vi "APC_9056_NI9214conf.vi"() -> (5 "channels name out":string[](array[string])=["WF-TT-001", "O2-TT-001", "AR-TT-001", "NG-TT-001", "NGDI-TT-001", "WF-TT-002 ", "WF-TT-003", "WF-TT-004", "WF-TT-007", "PC-TT-001", "PC-TT-002", "PC-TT-003", "PC-TT-004", "PC-TT-005", "PC-TT-006", "EC-TT-001", "EC-TT-002", "SW-TT-001", "SW-TT-002", "SW-TT-003", "SW-TT-004", "SW-TT-005", "SW-TT-006", "SW-TT-007", "SW-TT-008", "SW-TT-009", "EO-TT-001", "EO-TT-002", "NI9214b_13", "NI9214b_14", "NI9214b_15", "NI9214b_16"])   [LabVIEW 2020]
panel:
  in  "NI9214_B":string[](array[string])=["EC-TT-002", "SW-TT-001", "SW-TT-002", "SW-TT-003", "SW-TT-004", "SW-TT-005", "SW-TT-006", "SW-TT-007", "SW-TT-008", "SW-TT-009", "EO-TT-001", "EO-TT-002", "NI9214b_13", "NI9214b_14", "NI9214b_15", "NI9214b_16"]
  in  "NI9214_A":string[](array[string])=["WF-TT-001", "O2-TT-001", "AR-TT-001", "NG-TT-001", "NGDI-TT-001", "WF-TT-002 ", "WF-TT-003", "WF-TT-004", "WF-TT-007", "PC-TT-001", "PC-TT-002", "PC-TT-003", "PC-TT-004", "PC-TT-005", "PC-TT-006", "EC-TT-001"]
  # "NI9214"
  # "_degC is added automatically to all channels"
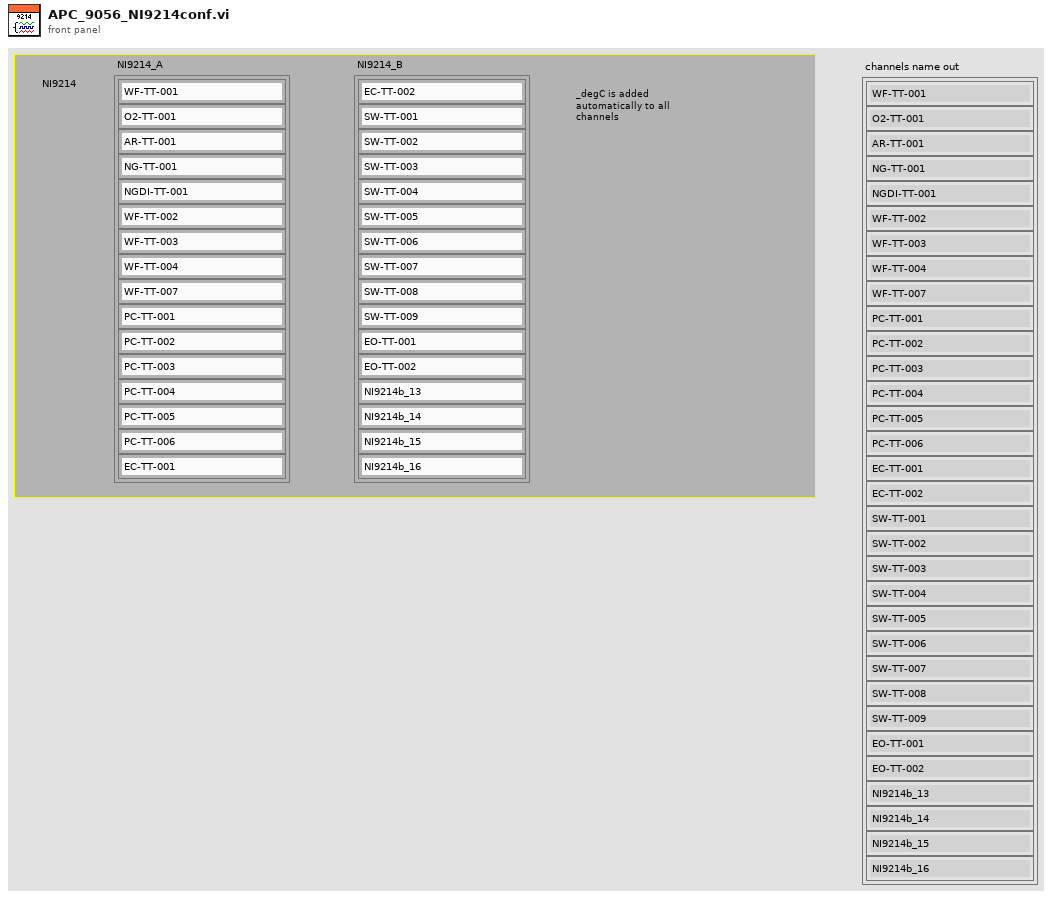
[diagram p1: front panel]
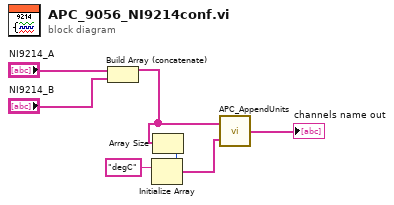
[diagram p0: block diagram]
diagram:
  n1 = Build Array (concatenate)("NI9214_A", "NI9214_B") -> (w3:string[])
  n2 = Array Size(array=w3) -> (size(s)=w4:i32)
  n3 = Initialize Array("degC" ("name to assign"), w4) -> (w2:string[])
  n4 = call "APC_AppendUnits.vi"("units"=w2, "names"=w3) -> ("names_units"=→"channels name out":string[])
